vi "Init Tunnel References.vi"(8 "error in (no error)":errorcluster, 11 "CSM-Helper in":refnum<class "CSM-Helper.lvclass">) -> (0 "error out":errorcluster, 3 "CSM-Helper out":refnum<class "CSM-Helper.lvclass">)   [LabVIEW 2020, in "CSM-Helper.lvclass"]
uses:
  CSM-Helper.lvclass
  CSM-Helper.lvclass/CSM-Helper.ctl
  <vilib>/Utility/Data Type/Type Definitions/Data Type.ctl
  <vilib>/Utility/Data Type/Type Definitions/Refnum Type.ctl
  <vilib>/Utility/Data Type/NI_Data Type.lvlib
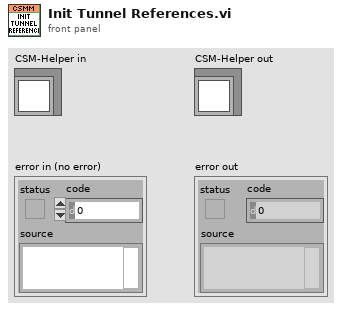
[diagram p1: front panel]
types:
  T1 = cluster{refnum<vi>, "Outer Term":refnum<vi>, "Data Type":variant, "Wire":refnum<vi>}
  T2 = typedef "NI_Data Type.lvlib/Data Type.ctl" = enum8{"Invalid Type", "Void", "I8", "I16", "I32", "I64", "U8", "U16", "U32", "U64", "Single Float", "Double Float", "Extended Float", "Single Complex", "Double Complex", "Extended Complex", "Enum U8", "Enum U16", "Enum U32", "Enum U64", "Single Float With Unit", "Double Float With Unit", "Extended Float With Unit", "Single Complex with Unit", "Double Complex with Unit", "Extended Complex with Unit", "Boolean", "String", "Path", "Picture", "Tag", "Array", "Cluster", "Variant", "LV Variant", "Waveform", "Timestamp", "Digital Waveform", "Digital Data", "ExpressData", "Refnum", "External Data", "VI", "Poly VI", "LabVIEW Class Instance", "Fixed Point", "Set Collection", "Map Collection"}
  T3 = typedef "NI_Data Type.lvlib/Type Definition Info.ctl" = cluster{"Name":string, "Timestamp":u32}
  T4 = typedef "NI_Data Type.lvlib/Refnum Type.ctl" = enum16{"NotARefnum", "UnknownRefnum", "Generic", "Datalog", "ByteStream", "Device", "Occurence", "TCPNetConnection", "Auto", "Menu", "Imaq", "Hardware", "DataSocket", "Visa", "IVI", "UDPNetConnection", "Notifier", "Queue", "Irda", "EventReg", "DotNet", "UserEvent", "Callback", "UNUSED_EMPTY_POSITION", "BlueToothNetConnection", "LVObjApp", "LVObjVI", "LVObjUnknown", "GenericClass", "UserDefinedRefnumTag", "DataValue", "RT FIFO", "TDMS File", "PythonSessionRefnum"}
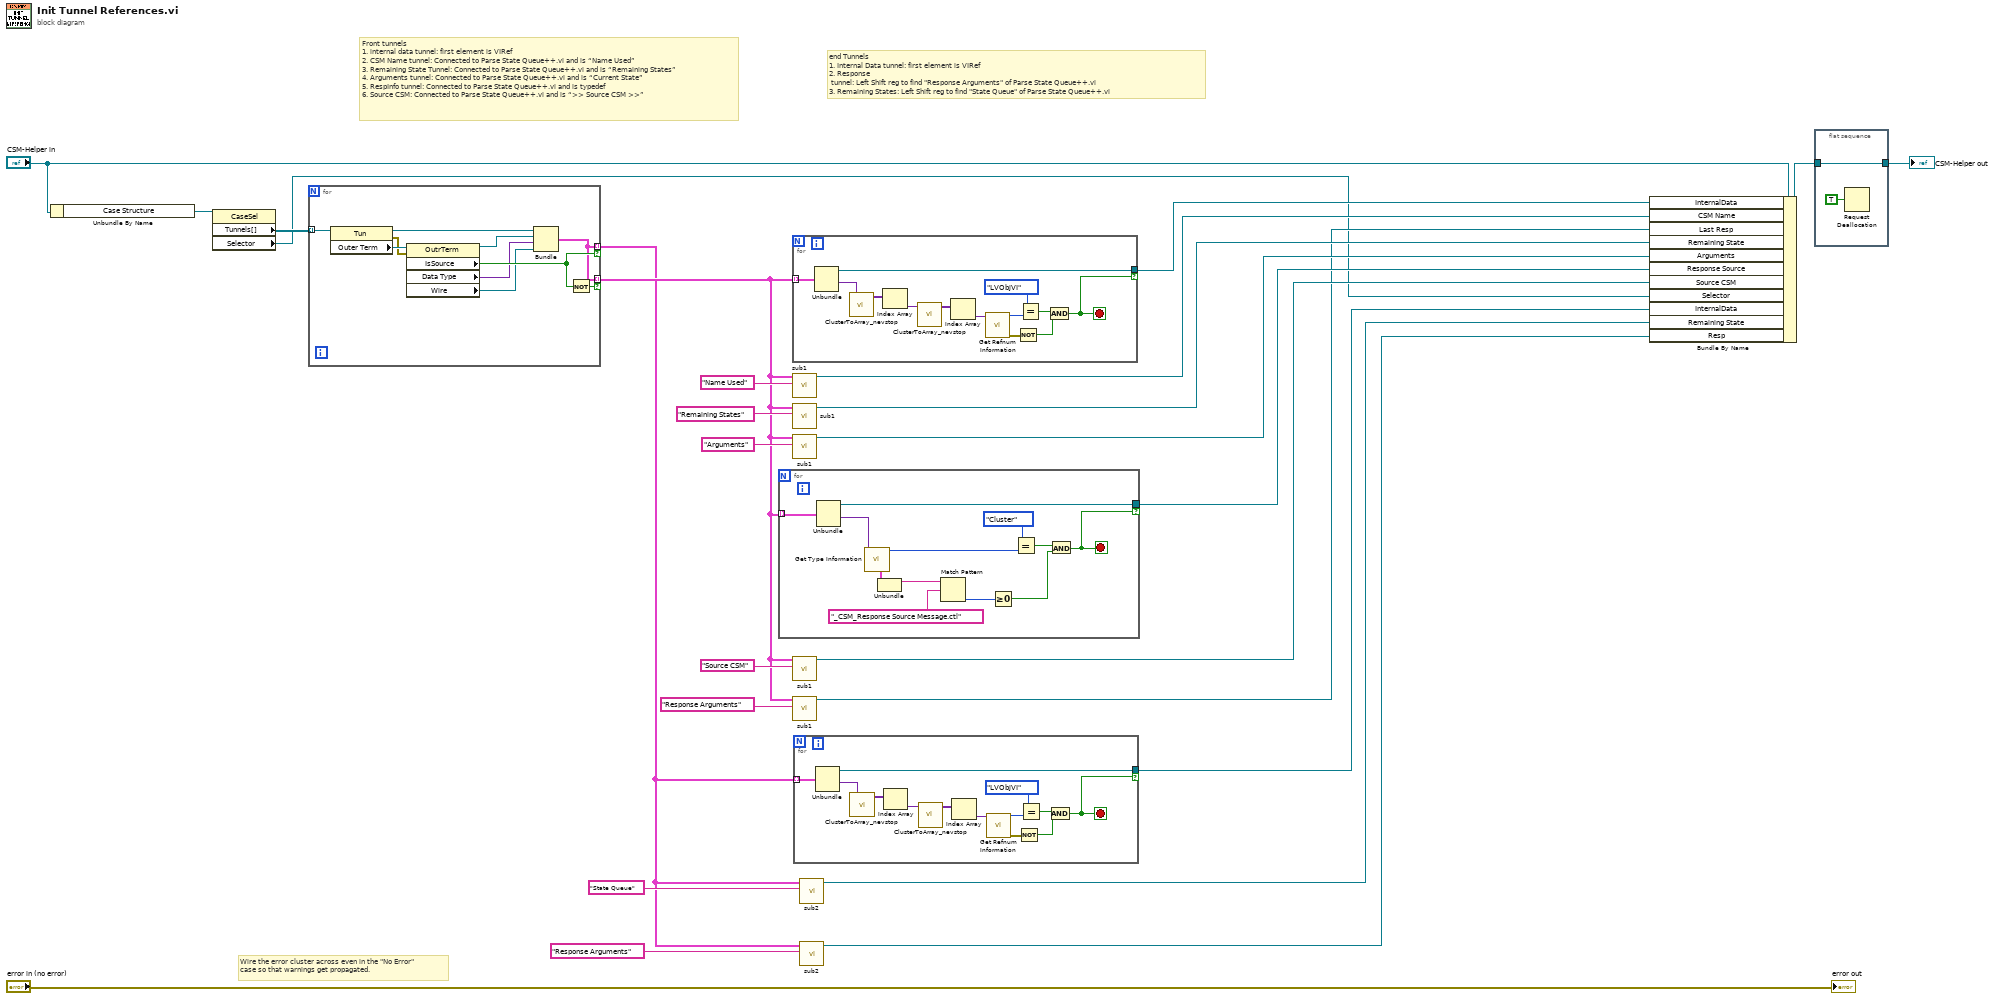
[diagram p0: block diagram]
diagram:
  # "end Tunnels\n1. Internal Data tunnel: first element is VIRef\n2. Response\n tunnel: Left Shift reg to find \"Response Arguments\" of Parse State Queue++.vi \n3. Remaining States: Left Shift reg to find \"State Queue\" of Parse State Queue++.vi"
  # "Front tunnels\n1. internal data tunnel: first element is VIRef\n2. CSM Name tunnel: Connected to Parse State Queue++.vi and is “Name Used”\n3. Remaining State Tunnel: Connected to Parse State Queue++.vi and is “Remaining States”\n4. Arguments tunnel: Connected to Parse State Queue++.vi and is “Current State”\n5. RespInfo tunnel: Connected to Parse State Queue++.vi and is typedef\n6. Source CSM: Connected to Parse State Queue++.vi and is “>> Source CSM >>”"
  # "Wire the error cluster across even in the \"No Error\"\ncase so that warnings get propagated."
  n1 = Unbundle By Name("CSM-Helper in") -> ("Case Structure"=w24:refnum<vi>)
  n2 = property class="CaseSel"(reference=w24) -> ("Tunnels[]"=w23:refnum<vi>[], "Selector"=w9:refnum<vi>)  [unwired: 1 in, 2 out]
  n3 = for {
    tunnel: w23 -> [w36] mode=indexing
    tunnel: [w29] -> w3 mode=indexing if=w33
    tunnel: [w29] -> w12 mode=indexing if=w32
    n4 = property class="Tun"(reference=w36) -> (reference out=w31:refnum<vi>, error out=w34:errorcluster, "Outer Term"=w35:refnum<vi>)  [unwired: 1 in]
    n5 = property class="OutrTerm"(reference=w35, error in=w34) -> (reference out=w30:refnum<vi>, "IsSource"=w33:bool, "Data Type"=w28:variant, "Wire"=w27:refnum<vi>)  [unwired: 1 out]
    n6 = Bundle(w31, "Outer Term"=w30, "Data Type"=w28, "Wire"=w27) -> (w29:T1)  [unwired: 1 in]
    n7 = Not(x=w33) -> (.not. x?=w32:bool)
  }
  n8 = for {
    tunnel: w12 -> [w48] mode=indexing
    tunnel: [w45] -> w13 if=w44
    stop <- w44 stop-if-true
    n9 = Unbundle(w48) -> (w45:refnum<vi>, "Data Type"=w41:variant)  [unwired: 2 out]
    n10 = call <vilib>:"Get Type Information.vi"("variant"=w41) -> ("type"=w47:T2, "type definition info"=w42:T3)  [unwired: 6 in, 3 out]
    n11 = Unbundle(w42) -> ("Name"=w40:string)  [unwired: 1 out]
    n12 = Match Pattern(string=w40, regular expression="_CSM_Response Source Message.ctl") -> (offset past match=w38:i32)  [unwired: 1 in, 3 out]
    n13 = Greater Or Equal To 0?(x=w38) -> (x >= 0?=w37:bool)
    n14 = Equal?(x=Data_Type."Cluster", y=w47) -> (x = y?=w46:bool)
    n15 = And(x=w46, y=w37) -> (x .and. y?=w44:bool)
  }
  n16 = for {
    tunnel: w12 -> [w61] mode=indexing
    tunnel: [w50] -> w22 if=w49
    stop <- w49 stop-if-true
    n17 = Unbundle(w61) -> (w50:refnum<vi>, "Data Type"=w60:variant)  [unwired: 2 out]
    n18 = call <userlib>:"ClusterToArray_nevstop.vi"("Cluster"=w60) -> ("Array"=w59:variant[])  [unwired: 10 in]
    n19 = Index Array(array=w59) -> (element=w58:variant)  [unwired: 1 in]
    n20 = call <userlib>:"ClusterToArray_nevstop.vi"("Cluster"=w58) -> ("Array"=w57:variant[])  [unwired: 10 in]
    n21 = Index Array(array=w57) -> (element=w56:variant)  [unwired: 1 in]
    n22 = call <vilib>:"Get Refnum Information.vi"("variant"=w56) -> ("error out"=w52:errorcluster, "reference type"=w54:T4)  [unwired: 7 in, 2 out]
    n23 = Not(x=w52) -> (.not. x?=w51:bool)
    n24 = Equal?(x=Refnum_Type."LVObjVI", y=w54) -> (x = y?=w53:bool)
    n25 = And(x=w53, y=w51) -> (x .and. y?=w49:bool)
  }
  n26 = call "sub1.vi"("regular expression"="Name Used", "Array"=w12) -> ("Tunnel out"=w21:refnum<vi>)  [unwired: 9 in]
  n27 = call "sub1.vi"("regular expression"="Remaining States", "Array"=w12) -> ("Tunnel out"=w18:refnum<vi>)  [unwired: 9 in]
  n28 = call "sub1.vi"("regular expression"="Arguments", "Array"=w12) -> ("Tunnel out"=w16:refnum<vi>)  [unwired: 9 in]
  n29 = call "sub1.vi"("regular expression"="Source CSM", "Array"=w12) -> ("Tunnel out"=w14:refnum<vi>)  [unwired: 9 in]
  n30 = call "sub1.vi"("regular expression"="Response Arguments", "Array"=w12) -> ("Tunnel out"=w10:refnum<vi>)  [unwired: 9 in]
  n31 = for {
    tunnel: w3 -> [w74] mode=indexing
    tunnel: [w63] -> w6 if=w62
    stop <- w62 stop-if-true
    n32 = Unbundle(w74) -> (w63:refnum<vi>, "Data Type"=w73:variant)  [unwired: 2 out]
    n33 = call <userlib>:"ClusterToArray_nevstop.vi"("Cluster"=w73) -> ("Array"=w72:variant[])  [unwired: 10 in]
    n34 = Index Array(array=w72) -> (element=w71:variant)  [unwired: 1 in]
    n35 = call <userlib>:"ClusterToArray_nevstop.vi"("Cluster"=w71) -> ("Array"=w70:variant[])  [unwired: 10 in]
    n36 = Index Array(array=w70) -> (element=w69:variant)  [unwired: 1 in]
    n37 = call <vilib>:"Get Refnum Information.vi"("variant"=w69) -> ("error out"=w65:errorcluster, "reference type"=w67:T4)  [unwired: 7 in, 2 out]
    n38 = Not(x=w65) -> (.not. x?=w64:bool)
    n39 = Equal?(x=Refnum_Type."LVObjVI", y=w67) -> (x = y?=w66:bool)
    n40 = And(x=w66, y=w64) -> (x .and. y?=w62:bool)
  }
  n41 = call "sub2.vi"("regular expression"="State Queue", "Array"=w3) -> ("Tunnel out"=w4:refnum<vi>)  [unwired: 9 in]
  n42 = call "sub2.vi"("regular expression"="Response Arguments", "Array"=w3) -> ("Tunnel out"=w1:refnum<vi>)  [unwired: 9 in]
  n43 = Bundle By Name(cluster="CSM-Helper in", "InternalData"=w22, "CSM Name"=w21, "Last Resp"=w10, "Remaining State"=w18, "Arguments"=w16, "Response Source"=w13, "Source CSM"=w14, "Selector"=w9, "InternalData"=w6, "Remaining State"=w4, "Resp"=w1) -> (w8:refnum<class "CSM-Helper.lvclass">)
  n44 = flat-sequence {
    tunnel: w8 -> [w75]
    tunnel: [w75] -> w7
    frame #0 {
      n45 = Request Deallocation(TRUE ("flag")) -> ()
    }
  }
  "error out" <- "error in (no error)"
  "CSM-Helper out" <- w7
